vi "UHR-Fleezers Control (host) - 11.0.vi"() -> ()   [LabVIEW 2011] (continued)
            w1289 = FALSE ("Value (Signaling)")
            n927 = case shown="True" w1288 {
              frame False {
              }
              frame True {
                n928 = property on="Sample Channel\nFlow" class="Bool (strict)"("Val(Sgnl)"=FALSE ("Stage Moving")) -> ()  [unwired: 2 in, 2 out]
              }
            }
            n929 = property on="Trap 1 (ON/OFF)" class="Bool (strict)"("Val(Sgnl)"=w1289) -> ()  [unwired: 2 in, 2 out]
            n930 = property on="Trap 2 (ON/OFF)" class="Bool (strict)"("Val(Sgnl)"=w1289) -> ()  [unwired: 2 in, 2 out]
            n931 = call <vilib>:"Beep.vi"() -> ()  [unwired: 3 in, 9 out]
          }
          frame #5 {
            n932 = property on="Move Cap. 2 (ADig Top)" class="Bool (strict)"("Val(Sgnl)"=TRUE ("Value (Signaling)")) -> ()  [unwired: 2 in, 2 out]
            n933 = property on="Tab Control" class="TabCtl (strict)"("Val(Sgnl)"=T4."Status" ("Value (Signaling)")) -> ()  [unwired: 2 in, 2 out]
          }
        }
      }
      event "Dip for Protein": Value Change {
        n934 = event-data() -> ()  [unwired: 1 in, 5 out]
        n935 = case shown="True" "Dip for Protein" {
          tunnel: w1295 -> [_ w1297]
          tunnel: w1294 -> [_ w1296]
          frame False {
          }
          frame True {
            n936 = while {
              tunnel: w1297 -> [w1308]
              tunnel: w1296 -> [w1307]
              i -> [w1302]
              stop <- w1304 stop-if-true
              n937 = Increment(x=w1302) -> (x+1=→"Dip #":i32)
              n938 = flat-sequence {
                tunnel: w1307 -> [w1319]
                tunnel: w1308 -> [w1320]
                tunnel: [w1320] -> w1312
                tunnel: [w1319] -> w1311
                tunnel: [w1313] -> w1298
                tunnel: [w1325] -> w1306
                tunnel: [w1326] -> w1305
                tunnel: w1312 -> [w1327]
                tunnel: w1311 -> [w1328]
                tunnel: [w1323] -> w1299
                tunnel: w1298 -> [w1323]
                tunnel: [w1336] -> w1310
                tunnel: w1306 -> [w1336]
                tunnel: [w1335] -> w1309
                tunnel: w1305 -> [w1335]
                tunnel: [w1332] -> w1303
                tunnel: [w1331] -> w1300
                tunnel: w1299 -> [w1331]
                tunnel: w1309 -> [w1356]
                tunnel: w1310 -> [w1357]
                tunnel: w1303 -> [w1358]
                tunnel: w1300 -> [w1355]
                tunnel: [w1414] -> w1304
                frame #0 {
                  n939 = local read "Trap Pos. FB ON"() -> (w1313:bool)
                  n940 = Compound Arithmetic op=AND("Flow ON\nduring dip?", "FB OFF when \nflow ON", w1313) -> (w1314:bool)
                  n941 = case shown="True" "Move trap \nbefore dip move?" {
                    frame False {
                    }
                    frame True {
                      n942 = property on="Trap Delta (MHz)" class="DigNum (strict)"("Val(Sgnl)"="Dipping Delta (MHz)") -> ()  [unwired: 2 in, 2 out]
                    }
                  }
                  n943 = property on="Green Laser ON/Interlacing" class="Bool (strict)"("Val(Sgnl)"="Green ON\nbefore dip?") -> ()  [unwired: 2 in, 2 out]
                  n944 = property on="Sample Channel\nFlow" class="Bool (strict)"("Val(Sgnl)"="Flow ON\nduring dip?") -> ()  [unwired: 2 in, 2 out]
                  n945 = case shown="True" w1314 {
                    frame False {
                    }
                    frame True {
                      n946 = property on="Trap Pos. FB ON" class="Bool (strict)"("Val(Sgnl)"=FALSE ("Value (Signaling)")) -> ()  [unwired: 2 in, 2 out]
                    }
                  }
                }
                frame #1 {
                  n947 = local read "Saved Stage Positions"() -> (w1330:dbl[][])
                  n948 = local write "Cancel dwell"(FALSE ("Cancel dwell")) -> ()
                  n949 = call "move to saved stage position.vi"("error in"=w1328, "Stage VISA resource name in"=w1327, "Position"="Dip Stage \nPosition", "Saved Stage Positions"=w1330) -> ("VISA resource name out"=w1325:refnum<visa-resource-name>, "error out"=w1326:errorcluster)
                }
                frame #2 {
                  n950 = node-c288() -> (w1334:T21)  [unwired: 4 in]
                  n951 = timed-loop {
                    timing: w1334 -> [_]
                    timing-out: [_] -> w1333
                    tunnel: [w1340] -> w1332
                    i -> [w1337]
                    stop <- w1341 stop-if-true
                    n952 = node-c288() -> ()  [unwired: 1 in, 1 out]
                    n953 = Greater Or Equal?(x=w1337, y="Dip Duration (s)") -> (x >= y?=w1349:bool)
                    n954 = local read "Dip for Protein"() -> (w1342:bool)
                    n955 = local read "Dump Beads"() -> (w1339:bool)
                    n956 = local read "Cancel dwell"() -> (w1348:bool)
                    n957 = local read "Pause dwell"() -> (w1345:bool)
                    n958 = Not(x=w1342) -> (.not. x?=w1347:bool)
                    n959 = Compound Arithmetic op=OR(w1348, w1349, w1347) -> (w1346:bool)
                    n960 = Select(t=FALSE, s=w1345, f=w1346) -> (s? t:f=w1343:bool)
                    n961 = Not(x=w1339) -> (.not. x?=w1338:bool)
                    n962 = node-c288() -> ()  [unwired: 1 in, 1 out]
                    n963 = And(x=w1342, y=w1338) -> (x .and. y?=w1340:bool)
                    n964 = Or(x=w1343, y=w1339) -> (x .or. y?=w1341:bool)
                    "Dip Time (s)" <- w1337
                  }
                  n965 = node-c288(w1333) -> ()  [unwired: 1 out]
                }
                frame #3 {
                  n966 = case shown="True" w1358 {
                    tunnel: w1357 -> [_ w1363]
                    tunnel: w1356 -> [_ w1362]
                    tunnel: w1355 -> [_ w1359]
                    frame False {
                    }
                    frame True {
                      n967 = flat-sequence {
                        tunnel: w1362 -> [w1367]
                        tunnel: w1363 -> [w1368]
                        tunnel: [w1368] -> w1361
                        tunnel: [w1367] -> w1360
                        tunnel: w1359 -> [w1364]
                        tunnel: w1361 -> [w1378]
                        tunnel: w1360 -> [w1377]
                        tunnel: w1359 -> [w1386]
                        frame #0 {
                          n968 = local read "Sample Channel\nFlow"() -> (w1366:bool)
                          n969 = case shown="True" w1366 {
                            tunnel: "Flow ON \nduring return\nfrom dip?" -> [w1369 w1372]
                            tunnel: w1364 -> [_ w1371]
                            frame False {
                              n970 = case shown="True" w1369 {
                                frame False {
                                }
                                frame True {
                                n971 = property on="Sample Channel\nFlow" class="Bool (strict)"("Val(Sgnl)"=TRUE ("Value (Signaling)")) -> ()  [unwired: 2 in, 2 out]
                                }
                              }
                            }
                            frame True {
                              n972 = case shown="False" w1372 {
                                tunnel: w1371 -> [w1373 _]
                                frame False {
                                n973 = property on="Trap Pos. FB ON" class="Bool (strict)"("Val(Sgnl)"=w1373) -> ()  [unwired: 2 in, 2 out]
                                n974 = property on="Sample Channel\nFlow" class="Bool (strict)"("Val(Sgnl)"=FALSE ("Value (Signaling)")) -> ()  [unwired: 2 in, 2 out]
                                }
                                frame True {
                                }
                              }
                            }
                          }
                        }
                        frame #1 {
                          # "For turning on green laser before stage reaches lower spot"
                          n975 = case shown="True" "Green ON\nafter start\nreturn?" {
                            frame False {
                            }
                            frame True {
                              n976 = flat-sequence {
                                frame #0 {
                                n977 = Multiply(x="Green delay after \nstart return (s)", y=1000.0) -> (x*y=w1383:dbl)
                                n978 = Wait (ms)(milliseconds to wait=w1383) -> ()  [unwired: 1 out]
                                }
                                frame #1 {
                                n979 = property on="Green Laser ON/Interlacing" class="Bool (strict)"("Val(Sgnl)"=TRUE ("Value (Signaling)")) -> ()  [unwired: 2 in, 2 out]
                                }
                              }
                            }
                          }
                          n980 = local read "Saved Stage Positions"() -> (w1381:dbl[][])
                          n981 = local write "Cancel dwell"(FALSE ("Cancel dwell")) -> ()
                          n982 = call "move to saved stage position.vi"("error in"=w1377, "Stage VISA resource name in"=w1378, "Position"="Return Stage \nPosition", "Saved Stage Positions"=w1381) -> ("error out"=w1379:errorcluster)  [unwired: 1 out]
                          n983 = local write "Stage Control Serial Error"(w1379) -> ()
                        }
                        frame #2 {
                          n984 = property on="Trap Pos. FB ON" class="Bool (strict)"("Val(Sgnl)"=w1386) -> ()  [unwired: 2 in, 2 out]
                          n985 = case shown="True" "Green ON \nafter return?" {
                            frame False {
                            }
                            frame True {
                              n986 = property on="Green Laser ON/Interlacing" class="Bool (strict)"("Val(Sgnl)"=TRUE ("Value (Signaling)")) -> ()  [unwired: 2 in, 2 out]
                            }
                          }
                          n987 = case shown="True" "Move trap after return?" {
                            frame False {
                            }
                            frame True {
                              n988 = property on="Trap Delta (MHz)" class="DigNum (strict)"("Val(Sgnl)"="Dip Trap Delta 2 (MHz)") -> ()  [unwired: 2 in, 2 out]
                            }
                          }
                          n989 = case shown="True" "Save data after return?" {
                            frame False {
                            }
                            frame True {
                              n990 = property on="Start Saving" class="Bool (strict)"("Val(Sgnl)"=TRUE ("Value (Signaling)")) -> ()  [unwired: 2 in, 2 out]
                            }
                          }
                          n991 = property on="Sample Channel\nFlow" class="Bool (strict)"("Val(Sgnl)"="Flow ON\nduring daq?") -> ()  [unwired: 2 in, 2 out]
                        }
                        frame #3 {
                          n992 = node-c288() -> (w1395:T21)  [unwired: 4 in]
                          n993 = timed-loop {
                            timing: w1395 -> [_]
                            timing-out: [_] -> w1394
                            i -> [w1396]
                            stop <- w1398 stop-if-true
                            n994 = node-c288() -> ()  [unwired: 1 in, 1 out]
                            n995 = local read "Dump Beads"() -> (w1397:bool)
                            n996 = Greater Or Equal?(x=w1396, y="Dwell Duration (s)") -> (x >= y?=w1403:bool)
                            n997 = local read "Dip for Protein"() -> (w1400:bool)
                            n998 = Not(x=w1400) -> (.not. x?=w1399:bool)
                            n999 = Compound Arithmetic op=OR(w1403, "Cancel dwell", w1399) -> (w1402:bool)
                            n1000 = node-c288() -> ()  [unwired: 1 in, 1 out]
                            n1001 = Select(t=FALSE, s="Pause dwell", f=w1402) -> (s? t:f=w1405:bool)
                            n1002 = Or(x=w1405, y=w1397) -> (x .or. y?=w1398:bool)
                            "Dwell Time (s)" <- w1396
                          }
                          n1003 = node-c288(w1394) -> ()  [unwired: 1 out]
                        }
                      }
                    }
                  }
                }
                frame #4 {
                  n1004 = local read "Dip for Protein"() -> (w1415:bool)
                  n1005 = local read "Dump Beads"() -> (w1412:bool)
                  n1006 = local write "Cancel dwell"(FALSE ("Cancel dwell")) -> ()
                  n1007 = Not(x=w1415) -> (.not. x?=w1416:bool)
                  n1008 = Not(x="Cont. Repeat Dipping?") -> (.not. x?=w1418:bool)
                  n1009 = Compound Arithmetic op=OR(w1416, w1418, w1412) -> (w1414:bool)
                }
              }
            }
          }
        }
      }
      event "Profile": Value Change {
        n1010 = event-data() -> ()  [unwired: 1 in, 5 out]
        n1011 = flat-sequence {
          tunnel: w1427 -> [w1430]
          tunnel: w1426 -> [w1438]
          tunnel: [w1432] -> w1425
          tunnel: [w1431] -> w1424
          tunnel: [w1429] -> w1422
          tunnel: [w1428] -> w1419
          tunnel: w1425 -> [w1445]
          tunnel: w1424 -> [w1444]
          tunnel: [w1442] -> w1423
          tunnel: w1422 -> [w1443]
          tunnel: [w1441] -> w1421
          tunnel: [w1440] -> w1420
          tunnel: w1419 -> [w1440]
          tunnel: w1423 -> [w1449]
          tunnel: w1421 -> [w1448]
          tunnel: w1420 -> [w1447]
          frame #0 {
            n1012 = call "Read Stage Position.vi"("error in"=w1438, "VISA resource name in"=w1430) -> ("Current Position"=w1428:cluster{dbl, dbl, dbl}, "error out"=w1431:errorcluster, "VISA resource name out"=w1429:refnum<visa-resource-name>)  [unwired: 1 out]
            "Current Position" <- w1428
            n1013 = local write "Stage Control Serial Error"(w1431) -> ()
            n1014 = Unbundle(w1428) -> (w1435:dbl, w1437:dbl, w1433:dbl)
            n1015 = Add(x=w1437, y="Y change (mm)") -> (x+y=w1434:dbl)
            n1016 = Bundle(w1435, w1434, w1433) -> (w1432:cluster{dbl, dbl, dbl})  [unwired: 1 in]
          }
          frame #1 {
            # "move to new position and start saving"
            n1017 = local write "Stage Moving"(TRUE ("Stage Moving")) -> ()
            n1018 = local write "Start Saving"(TRUE ("Start Saving")) -> ()
            n1019 = call "Set Stage Position.vi"("Position"=w1445, "error in"=w1444, "VISA resource name in"=w1443) -> ("error out"=w1441:errorcluster, "VISA resource name out"=w1442:refnum<visa-resource-name>)  [unwired: 1 out]
          }
          frame #2 {
            # "go back to start"
            n1020 = call "Set Stage Position.vi"("Position"=w1447, "error in"=w1448, "VISA resource name in"=w1449) -> ()  [unwired: 3 out]
          }
          frame #3 {
            # "stop saving"
            n1021 = local write "Stop Saving"(TRUE ("Stop Saving")) -> ()
            n1022 = local write "Stage Moving"(FALSE ("Stage Moving")) -> ()
          }
        }
      }
      event "Move to Position 1", "Move to Position 2", "Move to Position 3", "Move to Position 4", "Move to Position 5", "Lower Ch. Cap.": Value Change {
        n1023 = event-data() -> ()  [unwired: 1 in, 5 out]
        n1024 = Or(x="Move to Position 5", y="Lower Ch. Cap.") -> (x .or. y?=w1455:bool)
        n1025 = Build Array("Move to Position 1", "Move to Position 2", "Move to Position 3", "Move to Position 4", w1455) -> (w1458:bool[])
        n1026 = Boolean Array To Number(Boolean array=w1458) -> (number=w1457:u32)
        n1027 = Logarithm Base 2(1:w1457) -> (0:w1456:dbl)
        n1028 = flat-sequence {
          tunnel: w1456 -> [w1467]
          tunnel: w1453 -> [w1465]
          tunnel: w1452 -> [w1464]
          frame #0 {
            n1029 = local read "Saved Stage Positions"() -> (w1475:dbl[][])
            n1030 = Array Subset(array=w1475, index (row)=w1467, length (row)=1 ("length"), index (col)=1 ("index"), length (col)=3 ("length")) -> (w1472:dbl[][])
            n1031 = Reshape Array(w1472, 3 ("dimension size")) -> (w1470:dbl[])
            n1032 = Array To Cluster(array=w1470) -> (cluster=w1469:cluster{"[0]":dbl, "[1]":dbl, "[2]":dbl})
            n1033 = call "Set Stage Position.vi"("Position"=w1469, "error in"=w1464, "VISA resource name in"=w1465) -> ("error out"=w1468:errorcluster)  [unwired: 2 out]
            n1034 = local write "Stage Moving"(TRUE ("Stage Moving")) -> ()
            n1035 = local write "Stage Control Serial Error"(w1468) -> ()
          }
          frame #1 {
            n1036 = local write "Stage Moving"(FALSE ("Stage Moving")) -> ()
            n1037 = call <vilib>:"Beep.vi"() -> ()  [unwired: 3 in, 9 out]
          }
        }
      }
      event "Got ADig bead": Value Change {
        n1038 = event-data() -> ()  [unwired: 1 in, 5 out]
        n1039 = flat-sequence {
          frame #0 {
            n1040 = local read "Cap 1 Samp Flow ON"() -> (w1479:bool)
            n1041 = case shown="True" w1479 {
              frame False {
              }
              frame True {
                n1042 = property on="Sample Channel\nFlow" class="Bool (strict)"("Val(Sgnl)"=TRUE ("Value (Signaling)")) -> ()  [unwired: 2 in, 2 out]
              }
            }
          }
          frame #1 {
            n1043 = property on="Inject Pump 3" class="Bool (strict)"("Val(Sgnl)"=FALSE ("Value (Signaling)")) -> ()  [unwired: 2 in, 2 out]
          }
          frame #2 {
            n1044 = property on="Move Cap. 1 (DNA Bottom)" class="Bool (strict)"("Val(Sgnl)"=TRUE ("Value (Signaling)")) -> ()  [unwired: 2 in, 2 out]
          }
        }
      }
      event "Force FB Data\nScript": Value Change {
        n1045 = event-data() -> ()  [unwired: 1 in, 5 out]
        n1046 = flat-sequence {
          tunnel: w1488 -> [w1492]
          tunnel: w1489 -> [w1493]
          tunnel: [w1493] -> w1484
          tunnel: [w1492] -> w1483
          tunnel: w1484 -> [w1496]
          tunnel: w1483 -> [w1495]
          tunnel: ["Trap Trig Fl."] -> w1485
          tunnel: [w1521] -> w1486
          tunnel: w1485 -> [w1521]
          tunnel: [w1525] -> w1487
          tunnel: w1486 -> [w1525]
          tunnel: w1487 -> [w1527]
          frame #0 {
            n1047 = property on="Trap Delta (MHz)" class="DigNum (strict)"("Val(Sgnl)"="Trap Delta Before Moving") -> ()  [unwired: 2 in, 2 out]
          }
          frame #1 {
            n1048 = local read "Saved Stage Positions"() -> (w1498:dbl[][])
            n1049 = local write "FB Trap Pos Offset"(0.0 ("FB Trap Pos Offset")) -> ()
            n1050 = property on="Trap Pos. FB Offset Factor" class="DigNum (strict)"("Val(Sgnl)"=i64 0 ("Value (Signaling)")) -> ()  [unwired: 2 in, 2 out]
            n1051 = local write "Stage Moving"(TRUE ("Stage Moving")) -> ()
            n1052 = call "move to saved stage position.vi"("error in"=w1495, "Stage VISA resource name in"=w1496, "Position"="Stage Position To Establish FB", "Saved Stage Positions"=w1498) -> ("error out"=w1494:errorcluster)  [unwired: 1 out]
            n1053 = local write "Stage Control Serial Error"(w1494) -> ()
          }
          frame #2 {
            n1054 = call <vilib>:"Beep.vi"() -> ()  [unwired: 3 in, 9 out]
            n1055 = Multiply(x="Wait (s)", y=u32 1000 ("milliseconds to wait")) -> (x*y=w1504:u32)
            n1056 = property on="Trap Delta (MHz)" class="DigNum (strict)"("Val(Sgnl)"="Starting \nTrap Delta (MHz)") -> ()  [unwired: 2 in, 2 out]
            n1057 = local write "Stage Moving"(FALSE ("Stage Moving")) -> ()
            n1058 = Wait (ms)(milliseconds to wait=w1504) -> ()  [unwired: 1 out]
            n1059 = property on="Tab Control 2" class="TabCtl (strict)"("Val(Sgnl)"=T6."Feedback on Trap Position" ("Value (Signaling)")) -> ()  [unwired: 2 in, 2 out]
            n1060 = property on="Tab Control" class="TabCtl (strict)"("Val(Sgnl)"=T4."Trap Control (RF)" ("Value (Signaling)")) -> ()  [unwired: 2 in, 2 out]
          }
          frame #3 {
            n1061 = property on="Set Reading to\nSetpoint" class="Bool (strict)"("Val(Sgnl)"=TRUE ("Value (Signaling)")) -> ()  [unwired: 2 in, 2 out]
            n1062 = Wait (ms)(milliseconds to wait=u32 500) -> ()  [unwired: 1 out]
          }
          frame #4 {
            n1063 = property on="Trap Pos. FB ON" class="Bool (strict)"("Val(Sgnl)"=TRUE ("Value (Signaling)")) -> ()  [unwired: 2 in, 2 out]
            n1064 = Wait (ms)(milliseconds to wait=u32 250) -> ()  [unwired: 1 out]
          }
          frame #5 {
            n1065 = case shown="False" "Trap Trig Fl." {
              frame False {
                n1066 = case shown="True" "Green ON after FB ON?" {
                  selector: "Green ON after FB ON?" -> [_ w1520]
                  frame False {
                  }
                  frame True {
                    n1067 = property on="Green Laser ON/Interlacing" class="Bool (strict)"("Val(Sgnl)"=w1520) -> ()  [unwired: 2 in, 2 out]
                  }
                }
              }
              frame True {
              }
            }
            n1068 = case shown="True" "Remove Action Offset" {
              tunnel: TRUE ("Value (Signaling)") -> [w1517 w1518]
              frame False {
                n1069 = property on="Remove Unwinding Offset" class="Bool (strict)"("Val(Sgnl)"=w1517) -> ()  [unwired: 2 in, 2 out]
              }
              frame True {
                n1070 = property on="Remove Action Offset" class="Bool (strict)"("Val(Sgnl)"=w1518) -> ()  [unwired: 2 in, 2 out]
              }
            }
            n1071 = Wait (ms)(milliseconds to wait=u32 250) -> ()  [unwired: 1 out]
          }
          frame #6 {
            n1072 = property on="Start Saving" class="Bool (strict)"("Val(Sgnl)"=TRUE ("Value (Signaling)")) -> ()  [unwired: 2 in, 2 out]
            n1073 = Wait (ms)(milliseconds to wait=u32 5000) -> ()  [unwired: 1 out]
          }
          frame #7 {
            w1524 = TRUE ("Value (Signaling)")
            n1074 = property on="Rem fb disp offset" class="Bool (strict)"("Val(Sgnl)"=w1524) -> ()  [unwired: 2 in, 2 out]
            n1075 = property on="Remove Offset" class="Bool (strict)"("Val(Sgnl)"=w1524) -> ()  [unwired: 2 in, 2 out]
            n1076 = Wait (ms)(milliseconds to wait=u32 100) -> ()  [unwired: 1 out]
          }
          frame #8 {
            n1077 = case shown="True" w1527 {
              frame False {
              }
              frame True {
                n1078 = local write "Trap Trig. Fl."(TRUE ("Value (Signaling)")) -> ()
              }
            }
          }
          frame #9 {
            n1079 = case shown="True" "Start dipping after?" {
              frame False {
              }
              frame True {
                n1080 = flat-sequence {
                  frame #0 {
                    n1081 = Multiply(x="Delay before dipping (s)", y=1000.0) -> (x*y=w1531:dbl)
                    n1082 = Wait (ms)(milliseconds to wait=w1531) -> ()  [unwired: 1 out]
                  }
                  frame #1 {
                    n1083 = property on="Dip for Protein" class="Bool (strict)"("Val(Sgnl)"=TRUE ("Value (Signaling)")) -> ()  [unwired: 2 in, 2 out]
                    n1084 = local write "Scripts"(T1."Dipping" ("Scripts")) -> ()
                  }
                }
              }
            }
          }
        }
      }
      event "Fixed Traps Data\nScript": Value Change {
        n1085 = event-data() -> ()  [unwired: 1 in, 5 out]
        n1086 = flat-sequence {
          frame #0 {
            n1087 = case shown="True" "Green ON" {
              frame False {
              }
              frame True {
                n1088 = property on="Green Laser ON/Interlacing" class="Bool (strict)"("Val(Sgnl)"=TRUE) -> ()  [unwired: 2 in, 2 out]
              }
            }
            n1089 = local write "Offset (nm)"(0.0 ("Offset (nm)")) -> ()
            n1090 = property on="Sample Channel\nFlow" class="Bool (strict)"("Val(Sgnl)"=FALSE ("Value (Signaling)")) -> ()  [unwired: 2 in, 2 out]
            n1091 = property on="Trap Delta (MHz)" class="DigNum (strict)"("Val(Sgnl)"="Fixed Traps Trap Delta (MHz)") -> ()  [unwired: 2 in, 2 out]
          }
          frame #1 {
            n1092 = Wait (ms)(milliseconds to wait=u32 1000) -> ()  [unwired: 1 out]
          }
          frame #2 {
            n1093 = local write "Start Saving"(TRUE ("Start Saving")) -> ()
          }
          frame #3 {
            n1094 = local read "Bead Sep. Int. Time (s)"() -> (w1542:dbl)
            n1095 = Multiply(x=w1542, y=1000.0) -> (x*y=w1544:dbl)
            n1096 = Wait (ms)(milliseconds to wait=w1544) -> ()  [unwired: 1 out]
          }
          frame #4 {
            n1097 = property on="Remove Offset" class="Bool (strict)"("Val(Sgnl)"=TRUE ("Value (Signaling)")) -> ()  [unwired: 2 in, 2 out]
          }
          frame #5 {
            n1098 = property on="Dip for Protein" class="Bool (strict)"("Val(Sgnl)"="Start dipping after?") -> ()  [unwired: 2 in, 2 out]
          }
        }
      }
      event "Got DNA bead": Value Change {
        n1099 = event-data() -> ()  [unwired: 1 in, 5 out]
        n1100 = flat-sequence {
          frame #0 {
            n1101 = local read "Daq spot flow on"() -> (w1549:bool)
            n1102 = case shown="True" w1549 {
              frame False {
              }
              frame True {
                n1103 = property on="Sample Channel\nFlow" class="Bool (strict)"("Val(Sgnl)"=TRUE ("Value (Signaling)")) -> ()  [unwired: 2 in, 2 out]
              }
            }
            n1104 = property on="Got DNA bead" class="Bool"("Key Focus"=FALSE) -> ()  [unwired: 2 in, 2 out]
          }
          frame #1 {
            n1105 = property on="Inject Pump 1" class="Bool (strict)"("Val(Sgnl)"=FALSE ("Value (Signaling)")) -> ()  [unwired: 2 in, 2 out]
          }
          frame #2 {
            n1106 = property on="Cal/Data Acq. Spot" class="Bool (strict)"("Val(Sgnl)"=TRUE ("Value (Signaling)")) -> ()  [unwired: 2 in, 2 out]
          }
        }
      }
      event "Take Stepping Data": Value Change {
        n1107 = event-data() -> ()  [unwired: 1 in, 5 out]
        n1108 = local read "Save ave N"() -> (w1561:dbl)
        n1109 = flat-sequence {
          tunnel: w1561 -> [w1563]
          tunnel: [w1563] -> w1556
          tunnel: [w1565] -> w1557
          tunnel: w1556 -> [w1565]
          tunnel: [w1567] -> w1558
          tunnel: w1557 -> [w1567]
          tunnel: [w1570] -> w1559
          tunnel: w1558 -> [w1570]
          tunnel: [w1572] -> w1560
          tunnel: w1559 -> [w1572]
          tunnel: [w1574] -> w1554
          tunnel: w1560 -> [w1574]
          tunnel: w1554 -> [w1577]
          tunnel: [w1577] -> w1553
          tunnel: w1553 -> [w1578]
          tunnel: [w1578] -> w1555
          tunnel: w1555 -> [w1584]
          frame #0 {
            n1110 = property on="Save ave N" class="DigNum (strict)"("Val(Sgnl)"="Save ave factor") -> ()  [unwired: 2 in, 2 out]
          }
          frame #1 {
            n1111 = Wait (ms)(milliseconds to wait=u32 100) -> ()  [unwired: 1 out]
          }
          frame #2 {
            n1112 = local read "Offset 2 Start (MHz)"() -> (w1569:dbl)
            n1113 = property on="Saved AOD Raster Scan Parameter Sets" class="Arr (strict)"("Index Values"=u32[] [2]) -> ()  [unwired: 2 in, 2 out]
            n1114 = property on="Trap Delta (MHz)" class="DigNum (strict)"("Val(Sgnl)"=w1569) -> ()  [unwired: 2 in, 2 out]
          }
          frame #3 {
            n1115 = property on="Load parameters" class="Bool (strict)"("Val(Sgnl)"=TRUE ("Value (Signaling)")) -> ()  [unwired: 2 in, 2 out]
          }
          frame #4 {
            n1116 = Wait (ms)(milliseconds to wait=u32 100) -> ()  [unwired: 1 out]
          }
          frame #5 {
            n1117 = property on="Trap Raster Scan" class="Bool (strict)"("Val(Sgnl)"=TRUE ("Value (Signaling)")) -> ()  [unwired: 2 in, 2 out]
          }
          frame #6 {
            n1118 = Wait (ms)(milliseconds to wait=u32 1000) -> ()  [unwired: 1 out]
          }
          frame #7 {
            n1119 = while {
              stop <- w1581 stop-if-true
              n1120 = local read "Raster Scanning..."() -> (w1583:bool)
              n1121 = local read "Saving..."() -> (w1582:bool)
              n1122 = Not(x=w1582) -> (.not. x?=w1579:bool)
              n1123 = Not(x=w1583) -> (.not. x?=w1580:bool)
              n1124 = And(x=w1580, y=w1579) -> (x .and. y?=w1581:bool)
            }
          }
          frame #8 {
            n1125 = property on="Save ave N" class="DigNum (strict)"("Val(Sgnl)"=w1584) -> ()  [unwired: 2 in, 2 out]
          }
        }
      }
      event "Step Size (nm)": Value Change {
        n1126 = event-data() -> ()  [unwired: 1 in, 5 out]
        n1127 = flat-sequence {
          frame #0 {
            n1128 = property on="Saved AOD Raster Scan Parameter Sets" class="Arr (strict)"("Index Values"=u32[] [1]) -> ()  [unwired: 2 in, 2 out]
          }
          frame #1 {
            n1129 = Multiply(x="N Steps", y="Step Size (nm)") -> (x*y=w1586:dbl)
            n1130 = property on="Scan Speed AOD (nm/s) 2" class="DigNum (strict)"("Value"="Step Size (nm)") -> ()  [unwired: 2 in, 2 out]
            n1131 = property on="Step Size AOD (nm) 2" class="DigNum (strict)"("Value"="Step Size (nm)") -> ()  [unwired: 2 in, 2 out]
            n1132 = property on="Scan Range AOD (nm) 2" class="DigNum (strict)"("Value"=w1586) -> ()  [unwired: 2 in, 2 out]
          }
        }
      }
      event "Take Detection Laser\nImage": Value Change {
        n1133 = event-data() -> ()  [unwired: 1 in, 5 out]
        n1134 = flat-sequence {
          tunnel: [w1614] -> w1604
          tunnel: [w1613] -> w1597
          tunnel: [w1612] -> w1589
          tunnel: [w1617] -> w1605
          tunnel: w1604 -> [w1617]
          tunnel: [w1616] -> w1598
          tunnel: w1597 -> [w1616]
          tunnel: [w1615] -> w1590
          tunnel: w1589 -> [w1615]
          tunnel: [w1621] -> w1606
          tunnel: w1605 -> [w1621]
          tunnel: [w1620] -> w1599
          tunnel: w1598 -> [w1620]
          tunnel: [w1619] -> w1591
          tunnel: w1590 -> [w1619]
          tunnel: [w1627] -> w1607
          tunnel: w1606 -> [w1627]
          tunnel: [w1626] -> w1600
          tunnel: w1599 -> [w1626]
          tunnel: [w1625] -> w1592
          tunnel: w1591 -> [w1625]
          tunnel: [w1631] -> w1608
          tunnel: w1607 -> [w1631]
          tunnel: [w1630] -> w1601
          tunnel: w1600 -> [w1630]
          tunnel: [w1629] -> w1593
          tunnel: w1592 -> [w1629]
          tunnel: [w1635] -> w1609
          tunnel: w1608 -> [w1635]
          tunnel: [w1634] -> w1602
          tunnel: w1601 -> [w1634]
          tunnel: [w1633] -> w1594
          tunnel: w1593 -> [w1633]
          tunnel: [w1639] -> w1610
          tunnel: w1609 -> [w1639]
          tunnel: [w1638] -> w1603
          tunnel: w1602 -> [w1638]
          tunnel: [w1637] -> w1595
          tunnel: w1594 -> [w1637]
          tunnel: w1610 -> [w1645]
          tunnel: w1603 -> [w1644]
          tunnel: [w1642] -> w1596
          tunnel: w1595 -> [w1642]
          tunnel: w1596 -> [w1646]
          frame #0 {
            n1135 = local read "Green Laser ON/Interlacing"() -> (w1614:bool)
            n1136 = local read "Green laser mode"() -> (w1613:enum32{"Laser ON", "Laser OFF", "Interlace"})
            n1137 = local read "Green FB On/Off"() -> (w1612:bool)
          }
          frame #1 {
            n1138 = property on="Green FB On/Off" class="Bool (strict)"("Val(Sgnl)"=FALSE ("Value (Signaling)")) -> ()  [unwired: 2 in, 2 out]
          }
          frame #2 {
            n1139 = property on="Green Laser ON/Interlacing" class="Bool (strict)"("Val(Sgnl)"=TRUE ("Value (Signaling)")) -> ()  [unwired: 2 in, 2 out]
            n1140 = property on="Flip Green Filter" class="Bool (strict)"("Val(Sgnl)"=TRUE ("Value (Signaling)")) -> ()  [unwired: 2 in, 2 out]
            n1141 = property on="Green laser mode" class="RadioBtnsControl (strict)"("Val(Sgnl)"=enum32{"Laser ON", "Laser OFF", "Interlace"}."Laser ON" ("Value (Signaling)")) -> ()  [unwired: 2 in, 2 out]
          }
          frame #3 {
            n1142 = Wait (ms)(milliseconds to wait=u32 500) -> ()  [unwired: 1 out]
          }
          frame #4 {
            n1143 = property on="Confocal Image" class="Bool (strict)"("Val(Sgnl)"=TRUE ("Value (Signaling)")) -> ()  [unwired: 2 in, 2 out]
          }
          frame #5 {
            n1144 = Wait (ms)(milliseconds to wait=u32 2000) -> ()  [unwired: 1 out]
          }
          frame #6 {
            n1145 = while {
              stop <- w1640 stop-if-true
              n1146 = local read "Saving..."() -> (w1641:bool)
              n1147 = Not(x=w1641) -> (.not. x?=w1640:bool)
            }
          }
          frame #7 {
            n1148 = property on="Flip Green Filter" class="Bool (strict)"("Val(Sgnl)"=TRUE ("Value (Signaling)")) -> ()  [unwired: 2 in, 2 out]
            n1149 = property on="Green Laser ON/Interlacing" class="Bool (strict)"("Val(Sgnl)"=w1645) -> ()  [unwired: 2 in, 2 out]
            n1150 = property on="Green laser mode" class="RadioBtnsControl (strict)"("Val(Sgnl)"=w1644) -> ()  [unwired: 2 in, 2 out]
          }
          frame #8 {
            n1151 = property on="Green FB On/Off" class="Bool (strict)"("Val(Sgnl)"=w1646) -> ()  [unwired: 2 in, 2 out]
          }
        }
      }
      event "Stop All": Value Change {
        n1152 = event-data() -> ()  [unwired: 1 in, 5 out]
        n1153 = local read "Stop All"() -> (w1647:bool)
      }
    }
    n1154 = node-c288() -> ()  [unwired: 1 in, 1 out]
  }
  n1155 = node-c288() -> (w94:T21)  [unwired: 4 out]
  n1156 = timed-loop "Control parameters (event loop)" {
    tunnel: w1 -> [w1656]
    shift-right: [w1655] -> _
    shift-left: errorcluster {"status"=FALSE, "code"=0, "source"=""} ("error out") -> [w1654]
    tunnel: [w1653] -> _
    timing: w92 -> [_]
    timing-out: [_] -> w91
    tunnel: w64 -> [w1652]
    tunnel: w5 -> [w1651]
    tunnel: w4 -> [w1650]
    tunnel: w3 -> [w1649]
    tunnel: w2 -> [w1648]
    stop <- w1653 stop-if-true
    n1157 = node-c288() -> ()  [unwired: 2 out]
    n1158 = event shown="[20] \"Green laser mode\", \"Green Laser ON/Interlacing\": Value Change" {
      selector: _ -> [_ _ _ _ _ _ _ _ _ _ _ _ _ _ _ _ _ _ _ _ _ _ _ _ _ _ _ _ _ _ _ _ _ _ _ _ _ _ _ _ _ _ _ _ _ _ _ _ _ _ _ _ _ _ _ _ _ _ _ _ _ _ _ _ _ _ _ _ _ _ _ _ _ _ _]
      dyn-events: _ -> [_ _ _ _ _ _ _ _ _ _ _ _ _ _ _ _ _ _ _ _ _ _ _ _ _ _ _ _ _ _ _ _ _ _ _ _ _ _ _ _ _ _ _ _ _ _ _ _ _ _ _ _ _ _ _ _ _ _ _ _ _ _ _ _ _ _ _ _ _ _ _ _ _ _ _]
      timeout: _ -> [_ _ _ _ _ _ _ _ _ _ _ _ _ _ _ _ _ _ _ _ _ _ _ _ _ _ _ _ _ _ _ _ _ _ _ _ _ _ _ _ _ _ _ _ _ _ _ _ _ _ _ _ _ _ _ _ _ _ _ _ _ _ _ _ _ _ _ _ _ _ _ _ _ _ _]
      tunnel: w1656 -> [w1694 _ _ _ w1732 _ w1754 _ _ _ _ w1820 _ _ w1863 w1869 w1874 w1880 w1916 w1934 w1941 _ w1953 w1957 w1968 w1979 w1990 w2001 w2012 w2023 w2050 w2144 w2151 w2189 _ w2224 w2228 w2239 w2243 w2247 _ w2255 _ _ _ _ _ _ _ _ _ _ _ _ _ _ _ _ _ w2633 _ w2650 _ w2657 w2675 _ w2682 w2690 w2705 w2716 w2722 _ w2731 _ w2750]
      tunnel: [w1693 _ _ _ w1722 _ w1753 _ _ w1785 _ w1799 _ _ w1862 w1865 w1871 w1877 w1915 w1932 w1940 _ w1951 _ w1962 w1973 w1984 w1995 w2006 w2017 w2048 w2142 w2149 w2187 _ w2222 w2226 w2229 w2241 w2245 _ w2253 _ _ _ _ _ _ _ _ _ _ _ _ _ _ _ _ _ w2631 _ _ _ _ w2672 _ _ _ _ _ _ _ _ _ _] -> w1655
      tunnel: w1654 -> [w1692 _ _ _ w1731 _ w1752 _ _ w1785 _ w1819 _ _ w1861 w1864 w1870 w1876 w1914 w1933 w1939 _ w1952 w1956 w1967 w1978 w1989 w2000 w2011 w2022 w2049 w2143 w2150 w2188 _ w2223 w2227 w2238 w2242 w2246 _ w2254 _ _ _ _ _ _ _ _ _ _ _ _ _ _ _ _ _ w2632 _ w2649 _ w2656 w2674 _ w2681 w2689 w2704 w2715 w2721 _ w2730 _ w2749]
      tunnel: [_ _ _ _ _ _ _ _ _ w1784 _ _ _ _ _ _ _ _ _ _ _ _ _ _ _ _ _ _ _ _ _ _ _ _ _ _ _ _ _ _ _ _ _ _ _ _ _ _ _ _ _ _ _ _ _ _ _ _ _ _ _ _ _ _ _ _ _ _ _ _ _ _ _ _ _] -> w1653
      tunnel: [_ _ _ _ _ _ _ "Round T1 X" _ _ _ _ _ _ _ _ _ _ _ _ _ _ _ _ _ _ _ _ _ _ _ _ _ _ _ _ _ _ _ _ _ _ _ _ _ _ _ _ _ _ _ _ _ _ _ _ _ _ _ _ _ _ _ _ _ _ _ _ _ _ _ _ _ _ _] -> _
      tunnel: [_ _ _ "Adjust Scale\nto Mean" _ _ _ _ _ _ _ _ _ _ _ _ _ _ _ _ _ _ "Test ttrig" _ _ _ _ _ _ _ _ _ _ _ _ _ _ _ _ _ _ _ _ _ _ _ _ _ _ "Flush Sample" "Flush Pump 3" "Flush Pump 1" "Clear Volume" _ _ _ _ _ _ _ _ _ _ _ _ _ _ _ _ _ _ _ _ _ _] -> _
      tunnel: [_ _ _ _ _ _ _ _ "Round T2 X" _ "Delayed Interlace Start" _ _ _ _ _ _ _ _ _ _ _ _ _ _ _ _ _ _ _ _ _ _ _ _ _ _ _ _ _ _ _ _ _ _ _ _ _ _ _ _ _ _ _ _ _ _ _ _ _ _ _ _ _ _ _ _ _ _ _ _ _ _ _ _] -> _
      tunnel: w1652 -> [_ _ _ _ _ _ _ _ _ _ _ _ _ _ _ _ _ _ _ _ _ _ _ _ _ _ _ _ _ _ _ _ _ _ _ _ _ _ _ _ _ _ _ _ _ w2412 w2419 w2426 w2431 w2440 _ _ w2546 _ _ _ _ _ _ _ _ _ _ _ _ _ _ _ _ _ _ _ _ _ _]
      tunnel: w1651 -> [_ _ _ _ _ _ _ _ _ _ _ _ _ _ _ _ _ _ _ _ _ _ _ _ _ _ _ _ _ _ _ _ _ _ _ _ _ _ _ _ _ _ _ w2329 _ _ _ _ _ _ w2484 _ _ w2552 _ w2561 _ w2575 _ _ _ _ _ _ _ _ _ _ _ _ _ _ _ _ _]
      tunnel: w1650 -> [_ _ _ _ _ _ _ _ _ _ _ _ _ _ _ _ _ _ _ _ _ _ _ _ _ _ _ _ _ _ _ _ _ _ _ _ _ _ _ _ _ _ _ _ _ _ _ _ _ _ _ _ _ _ _ _ _ _ _ _ _ _ _ _ _ _ _ _ _ _ _ _ _ _ _]
      tunnel: w1649 -> [_ _ _ _ _ _ _ _ _ _ _ _ _ _ _ _ _ _ _ _ _ _ _ _ _ _ _ _ _ _ _ _ _ _ _ _ _ _ _ _ _ _ w2266 _ _ _ _ _ _ _ _ w2514 _ _ w2557 _ w2568 _ w2600 _ _ _ _ _ _ _ _ _ _ _ _ _ _ _ _]
      tunnel: w1648 -> [_ _ _ _ _ _ _ _ _ _ _ _ _ _ _ _ _ _ _ _ _ _ _ _ _ _ _ _ _ _ _ _ _ _ _ _ _ _ _ _ _ _ _ _ _ _ _ _ _ _ _ _ _ _ _ _ _ _ _ _ _ _ _ _ _ _ _ _ _ _ _ _ _ _ _]
      event "AI Count (ticks)", "Sets to FIFO (Traps)", "Save ave N", "FPGA Ave.", "# Samples/channel", "N sets to save": Value Change {
        # "So that if 'Save ave N' is updated, the AOD scanning code updates too."
        n1159 = event-data() -> ()  [unwired: 6 out]
        n1160 = local read "AI Count (ticks)"() -> (w1674:u32)
        n1161 = Boolean To (0,1)(Boolean="Sets to FIFO (Traps)") -> (0, 1=w1684:cluster{"Set 1":i16, "Set 2":i16, "Set 3":i16})
        n1162 = xnode "Read/Write Control"("FPGA VI Reference In"=w1694, "error in"=w1692, "ai count"=w1674, "AI1 Sets to FIFO"="Sets to FIFO (Traps)", "N of AI1 Int Acq Sets"="N Acq Sets (Traps + Fl.)") -> ("error out"=w1693:errorcluster)  [unwired: 1 out]
        n1163 = Cluster To Array(cluster=w1684) -> (array=w1683:i16[])
        n1164 = To Unsigned Long Integer(number=w1683) -> (unsigned 32bit integer=w1663:u32[])
        n1165 = local read "Scan steps (AOD)"() -> (w1685:u64)
        n1166 = Multiply(x=w1674, y="N Acq Sets (Traps + Fl.)") -> (x*y=w1672:u32)
        n1167 = Divide(x=40000000.0, y=w1674) -> (x/y=w1666:dbl)
        "AI rate (Hz)" <- w1666
        "Ave. Rate (Hz)" <- w1666
        n1168 = Add Array Elements(numeric array=w1663) -> (sum=w1675:u32)
        "Trap Sets" <- w1675
        n1169 = Reciprocal(x=w1666) -> (1/x=→"Ave. Period (s)":dbl)
        n1170 = property on="Scan steps (AOD)" class="DigNum (strict)"("Val(Sgnl)"=w1685) -> ()  [unwired: 2 in, 2 out]
        n1171 = Divide(x=w1666, y="N Acq Sets (Traps + Fl.)") -> (x/y=w1689:dbl)
        "Data Rate (Hz)" <- w1689
        n1172 = Reciprocal(x=w1689) -> (1/x=→"Data Period (s)":dbl)
        n1173 = local read "Save ave N"() -> (w1688:dbl)
        n1174 = Divide(x=w1689, y=w1688) -> (x/y=w1687:dbl)
        "Save Data Rate (Hz)" <- w1687
        n1175 = Reciprocal(x=w1687) -> (1/x=→"Save Data Period (s)":dbl)
        n1176 = Multiply(x=w1672, y="# Samples/trap") -> (x*y=w1670:u32)
        "Counts/DMA" <- w1670
        n1177 = property on="Trap Disp. Downsample" class="DigNum (strict)"("Maximum"="# Samples/trap") -> ()  [unwired: 2 in, 2 out]
        n1178 = Multiply(x=w1675, y="# Samples/trap") -> (x*y=w1664:u32)
        "# Samples/channel" <- w1664
        n1179 = Multiply(x=w1664, y=u32 8) -> (x*y=→"Trap AI Elements/DMA read":u32)
        n1180 = local read "APD Int. Count"() -> (w1671:u32)
        n1181 = Multiply(x=w1664, y=u32 3) -> (x*y=→"Trap Pos Elements/DMA read":u32)
        n1182 = Divide(x=w1670, y=w1671) -> (x/y=w1661:dbl)
        "APD Samples/FIFO Acq." <- w1661
        n1183 = Divide(x=w1670, y=40000000.0) -> (x/y=w1668:dbl)
        "DMA Update Period (s)" <- w1668
        n1184 = Multiply(x=2.0, y=w1661) -> (x*y=→"APD Elements/DMA read":dbl)
        n1185 = property on="APD Disp. Downsample" class="DigNum (strict)"("Maximum"=w1661) -> ()  [unwired: 2 in, 2 out]
        n1186 = local read "N sets to save"() -> (w1681:u32)
        n1187 = Multiply(x=w1668, y=w1681) -> (x*y=→"Total Time (s)":dbl)
        "FPGA Averaging" <- FALSE ("FPGA Averaging")
      }
      event "Remove Offset": Value Change {
        n1188 = event-data() -> ()  [unwired: 7 out]
        n1189 = local write "Remove Offset"(FALSE ("Remove Offset")) -> ()
        n1190 = local read "Bead Mean (nm)"() -> (w1696:dbl)
        n1191 = local read "Offset (nm)"() -> (w1697:dbl)
        n1192 = Add(x=w1696, y=w1697) -> (x+y=w1695:dbl)
        n1193 = local write "Offset (nm)"(w1695) -> ()
        n1194 = disable-structure shown="Disabled" {
          frame Disabled {
            n1195 = local read "Bead Mean (nm)"() -> (w1702:dbl)
            n1196 = Add(y=w1702) -> (x=w1701:dbl, x+y=w1700:dbl)
            n1197 = Subtract(x=w1702, y=w1701) -> (x-y=w1699:dbl)
            n1198 = property on="Bead Separation" class="WFChart (strict)"("YScale.Minimum"=w1699) -> ()  [unwired: 2 in, 2 out]
            n1199 = property on="Bead Separation" class="WFChart (strict)"("YScale.Maximum"=w1700) -> ()  [unwired: 2 in, 2 out]
          }
          frame Enabled {
          }
        }
      }
      event "Detector Type": Value Change {
        n1200 = event-data() -> ()  [unwired: 7 out]
        n1201 = local read "AI labels"() -> (w1703:string[])
        n1202 = property on="High Res. Display" class="Ring (strict)"("Strings []"=w1703) -> ()  [unwired: 2 in, 2 out]
        n1203 = Build Array (concatenate)(w1703, "none") -> (w1704:string[])
        n1204 = property on="FFT 1 Choice 1" class="Ring (strict)"("Strings []"=w1704) -> ()  [unwired: 2 in, 2 out]
        n1205 = property on="FFT 1 Choice 2" class="Ring (strict)"("Strings []"=w1704) -> ()  [unwired: 2 in, 2 out]
        n1206 = property on="FFT 2 Choice 1" class="Ring (strict)"("Strings []"=w1704) -> ()  [unwired: 2 in, 2 out]
        n1207 = property on="FFT 2 Choice 2" class="Ring (strict)"("Strings []"=w1704) -> ()  [unwired: 2 in, 2 out]
        n1208 = Bundle("APD 1", "APD 2") -> (w1707:cluster{string, string})  [unwired: 1 out]
        n1209 = Cluster To Array(cluster=w1707) -> (array=w1705:string[])
        n1210 = Build Array (concatenate)(w1705, w1704) -> (w1709:string[])
        n1211 = Array Size(array=w1709) -> (size(s)=w1710:i32)
        n1212 = property on="Signals to Plot" class="LstBox (strict)"("Item Names"=w1709) -> ()  [unwired: 2 in, 2 out]
        n1213 = property on="Signals to Plot" class="LstBox (strict)"("Number of Rows"=w1710) -> ()  [unwired: 2 in, 2 out]
        n1214 = property on="All Signals" class="WFChart (strict)"("LegNumRows"=w1710) -> ()  [unwired: 2 in, 2 out]
      }
      event "Adjust Scale\nto Mean": Value Change {
        n1215 = event-data() -> ()  [unwired: 7 out]
        n1216 = local read "APD 1 Rate (Hz)"() -> (w1719:dbl)
        n1217 = Multiply(x=1000.0, y="Above (kHz)") -> (x*y=w1717:dbl)
        n1218 = Multiply(x=1000.0, y="Below (kHz)") -> (x*y=w1715:dbl)
        n1219 = Add(x=w1717, y=w1719) -> (x+y=w1712:dbl)
        n1220 = Subtract(x=w1719, y=w1715) -> (x-y=w1713:dbl)
        n1221 = property on="APD Chart" class="WFChart (strict)"("YScale.Minimum"=w1713) -> ()  [unwired: 2 in, 2 out]
        n1222 = property on="APD Chart" class="WFChart (strict)"("YScale.Maximum"=w1712) -> ()  [unwired: 2 in, 2 out]
      }
      event "Phase adj. (AI1)", "+ phase (AI1)", "- phase (AI1)": Value Change {
        n1223 = event-data() -> ()  [unwired: 7 out]
        n1224 = Negate(x="Phase adj. (AI1)") -> (-x=w1729:i16)
        n1225 = Select(t=w1729, s="- phase (AI1)", f="Phase adj. (AI1)") -> (s? t:f=w1728:i16)
        n1226 = xnode "Read/Write Control"("FPGA VI Reference In"=w1732, "error in"=w1731, "Phase count adjustment"=w1728) -> ("FPGA VI Reference Out"=w1727:T19, "error out"=w1726:errorcluster)
        n1227 = Or(x="- phase (AI1)", y="+ phase (AI1)") -> (x .or. y?=w1723:bool)
        n1228 = xnode "Read/Write Control"("FPGA VI Reference In"=w1727, "error in"=w1726, "+ phase"=w1723) -> ("error out"=w1722:errorcluster)  [unwired: 1 out]
      }
      event "Signals to Plot": Double Click {
        w1735 = u32 9868950 ("Color Box")
        n1229 = event-data() -> ("Row"=w1737:i32)  [unwired: 9 out]
        n1230 = property on="All Signals" class="WFChart (strict)"("Active Plot"=w1737) -> (error out=w1748:errorcluster)  [unwired: 2 in, 1 out]
        n1231 = property on="All Signals" class="WFChart (strict)" props=["Plot", "Visible?", "Plot", "Plot Color"](error in=w1748) -> (error out=w1747:errorcluster, "Plot.Visible?"=w1746:bool)  [unwired: 1 in, 2 out]
        n1232 = Select(t=FALSE ("Plot.Visible"), s=w1746, f=TRUE ("Plot.Visible")) -> (s? t:f=w1741:bool)
        n1233 = property on="All Signals" class="WFChart (strict)"(error in=w1747, "Plot.Visible?"=w1741) -> (error out=w1743:errorcluster)  [unwired: 1 in, 1 out]
        n1234 = property on="All Signals" class="WFChart (strict)"(error in=w1743) -> (error out=w1738:errorcluster, "Plot.Plot Color"=w1742:u32)  [unwired: 1 in, 1 out]
        n1235 = property on="Signals to Plot" class="LstBox (strict)"(error in=w1738, "Active Row"=w1737) -> (error out=w1736:errorcluster)  [unwired: 1 in, 1 out]
        n1236 = Select(t=w1742, s=w1741, f=u32 0) -> (s? t:f=w1739:u32)
        n1237 = property on="Signals to Plot" class="LstBox (strict)"(error in=w1736, "CellFontColor"=w1739, "SelColor"=w1735, "CellBG"=w1735, "CellFontSize"=u32 20 ("Active Row:Cell Font:Size"), "CellFontBold"=TRUE ("Active Row:Cell Font:Bold")) -> ()  [unwired: 1 in, 2 out]
      }
      event "BD 1 Frequency 1 (MHz)", "BD 1 Frequency 2 (MHz)", "BD 1 Frequency 3 (MHz)", "BD 2 Frequency 1 (MHz)", "BD 2 Frequency 2 (MHz)", "BD 2 Frequency 3 (MHz)", "Trap Delta (MHz)": Value Change {
        n1238 = event-data() -> ("CtlRef"=w1751:refnum<vi>)  [unwired: 6 out]
        n1239 = control-ref of="Trap Delta (MHz)"() -> (w1750:refnum<vi>)
        n1240 = Equal?(x=w1750, y=w1751) -> (x = y?=w1749:bool)
        n1241 = case shown="False" "Oscillate Set 1" {
          tunnel: w1754 -> [w1774 _]
          tunnel: [w1773 w1777] -> w1753
          tunnel: w1752 -> [w1772 w1777]
          tunnel: w1749 -> [w1757 _]
          frame False {
            n1242 = local read "BD 1 Frequency 2 (MHz)"() -> (w1761:dbl)
            n1243 = local read "BD 1 Frequency 1 (MHz)"() -> (w1759:dbl)
            n1244 = Subtract(x=w1761, y="Trap Delta (MHz)") -> (x-y=w1758:dbl)
            n1245 = Select(t=w1758, s=w1757, f=w1759) -> (s? t:f=w1756:dbl)
            n1246 = local read "Y RF Frequency Limits (MHz)"() -> (w1762:T16)
            n1247 = local read "X RF Frequency Limits (MHz)"() -> (w1763:T16)
            n1248 = local read "BD 1 Frequency 3 (MHz)"() -> (w1775:dbl)
            n1249 = local write "BD 1 Frequency 1 (MHz)"(w1756) -> ()
            n1250 = local read "BD 2 Frequency 1 (MHz)"() -> (w1766:dbl)
            n1251 = local read "BD 2 Frequency 2 (MHz)"() -> (w1765:dbl)
            n1252 = local read "BD 2 Frequency 3 (MHz)"() -> (w1776:dbl)
            n1253 = call "set RF board frequency - interlace.vi"("Board 2 Frequency Limits"=w1762, "Board 1 Frequency Limits"=w1763, "error in"=w1772, "FPGA VI Reference In"=w1774, "Board 2 Frequency 3 (MHz)"=w1776, "Board 1 Frequency 3 (MHz)"=w1775, "Board 2 Frequency 2 (MHz)"=w1765, "Board 2 Frequency 1 (MHz)"=w1766, "Board 1 Frequency 2 (MHz)"=w1761, "Board 1 Frequency 1  (MHz)"=w1756) -> ("error out"=w1773:errorcluster)  [unwired: 1 out]
            n1254 = Subtract(x=w1766, y=w1765) -> (x-y=w1770:dbl)
            n1255 = Subtract(x=w1756, y=w1761) -> (x-y=w1771:dbl)
            n1256 = Square(x=w1770) -> (x^2=w1768:dbl)
            n1257 = Square(x=w1771) -> (x^2=w1769:dbl)
            n1258 = Add(x=w1769, y=w1768) -> (x+y=w1767:dbl)
            n1259 = Square Root(x=w1767) -> (sqrt(x)=w1764:dbl)
            n1260 = local write "Trap Delta (MHz)"(w1764) -> ()
            n1261 = property on="Initial delta (MHz)" class="DigNum (strict)"("Val(Sgnl)"=w1764) -> ()  [unwired: 2 in, 2 out]
          }
          frame True {
          }
        }
      }
      event "Round T1 X": Value Change {
        n1262 = event-data() -> ()  [unwired: 7 out]
        n1263 = local read "BD 1 Frequency 1 (MHz)"() -> (w1780:dbl)
        n1264 = Round To Nearest(number=w1780) -> (nearest integer value=w1779:dbl)
        n1265 = property on="BD 1 Frequency 1 (MHz)" class="DigNum (strict)"("Val(Sgnl)"=w1779) -> ()  [unwired: 2 in, 2 out]
      }
      event "Round T2 X": Value Change {
        n1266 = event-data() -> ()  [unwired: 7 out]
        n1267 = local read "BD 1 Frequency 2 (MHz)"() -> (w1782:dbl)
        n1268 = Round To Nearest(number=w1782) -> (nearest integer value=w1781:dbl)
        n1269 = property on="BD 1 Frequency 2 (MHz)" class="DigNum (strict)"("Val(Sgnl)"=w1781) -> ()  [unwired: 2 in, 2 out]
      }
      event "Stop All": Value Change {
        n1270 = event-data() -> ()  [unwired: 7 out]
        n1271 = local read "Stop All"() -> (w1784:bool)
      }
      event "Delayed Interlace Start": Value Change {
        n1272 = event-data() -> ()  [unwired: 7 out]
        n1273 = flat-sequence {
          frame #0 {
            n1274 = Multiply(x="Delay to Interlace (s)", y=1000.0) -> (x*y=w1787:dbl)
            n1275 = Wait (ms)(milliseconds to wait=w1787) -> ()  [unwired: 1 out]
          }
          frame #1 {
            n1276 = property on="Green laser mode" class="RadioBtnsControl (strict)"("Val(Sgnl)"=enum32{"Laser ON", "Laser OFF", "Interlace"}."Interlace" ("Value (Signaling)")) -> ()  [unwired: 2 in, 2 out]
          }
        }
      }
      event "BD 1 Amplitude 1 (%)", "BD 1 Amplitude 2 (%)", "BD 1 Amplitude 3 (%)", "BD 2 Amplitude 1 (%)", "BD 2 Amplitude 2 (%)", "BD 2 Amplitude 3 (%)", "Trap 1 ON", "Trap 2 ON", "Trap 3 ON", "Feedback On/Off", "All FB On/Off": Value Change {
        w1811 = i16 1 ("f")
        n1277 = event-data() -> ()  [unwired: 7 out]
        n1278 = local write "Trap 1 (ON/OFF)"("Trap 1 ON") -> ()
        n1279 = local write "Trap 2 (ON/OFF)"("Trap 2 ON") -> ()
        n1280 = Boolean To (0,1)(Boolean="Trap 3 ON") -> (0, 1=w1812:i16)
        n1281 = Boolean To (0,1)(Boolean="Trap 1 ON") -> (0, 1=w1813:i16)
        n1282 = Boolean To (0,1)(Boolean="Trap 2 ON") -> (0, 1=w1814:i16)
        n1283 = Select(t=w1814, s="Trap ON/OFF X or Y Amp?", f=w1811) -> (s? t:f=w1809:i16)
        n1284 = Select(t=w1813, s="Trap ON/OFF X or Y Amp?", f=w1811) -> (s? t:f=w1810:i16)
        n1285 = Select(t=w1812, s="Trap ON/OFF X or Y Amp?", f=w1811) -> (s? t:f=w1808:i16)
        n1286 = Select(t=w1811, s="Trap ON/OFF X or Y Amp?", f=w1814) -> (s? t:f=w1806:i16)
        n1287 = Select(t=w1811, s="Trap ON/OFF X or Y Amp?", f=w1813) -> (s? t:f=w1807:i16)
        n1288 = Select(t=w1811, s="Trap ON/OFF X or Y Amp?", f=w1812) -> (s? t:f=w1805:i16)
        n1289 = And(x="All FB On/Off", y="Feedback On/Off") -> (x .and. y?=w1803:cluster{"Set 1":bool, "Set 2":bool})
        n1290 = local read "BD 1 Amplitude 1 (%)"() -> (w1823:dbl)
        n1291 = local read "BD 1 Amplitude 2 (%)"() -> (w1822:dbl)
        n1292 = local read "BD 1 Amplitude 3 (%)"() -> (w1821:dbl)
        n1293 = Unbundle By Name(w1803) -> ("Set 1"=w1798:bool, "Set 2"=w1795:bool)
        n1294 = local read "Y RF Amplitude Limits (%)"() -> (w1791:T16)
        n1295 = local read "X RF Amplitude Limits (%)"() -> (w1792:T16)
        n1296 = local read "BD 2 Amplitude 1 (%)"() -> (w1824:dbl)
        n1297 = local read "BD 2 Amplitude 2 (%)"() -> (w1825:dbl)
        n1298 = local read "BD 2 Amplitude 3 (%)"() -> (w1826:dbl)
        n1299 = And(x="Trap 2 ON", y=w1795) -> (x .and. y?=w1793:bool)
        n1300 = And(x="Trap 1 ON", y=w1798) -> (x .and. y?=w1796:bool)
        n1301 = Multiply(x=w1810, y=w1823) -> (x*y=w1818:dbl)
        n1302 = Multiply(x=w1822, y=w1809) -> (x*y=w1816:dbl)
        n1303 = Multiply(x=w1821, y=w1808) -> (x*y=w1817:dbl)
        n1304 = Multiply(x=w1824, y=w1807) -> (x*y=w1827:dbl)
        n1305 = Multiply(x=w1825, y=w1806) -> (x*y=w1828:dbl)
        n1306 = Multiply(x=w1826, y=w1805) -> (x*y=w1829:dbl)
        n1307 = call "set RF board amplitude - interlace.vi"("Board 2 Amplitude Limits"=w1791, "Board 1 Amplitude Limits"=w1792, "error in"=w1819, "FPGA VI Reference In"=w1820, "Board 2 Amplitude 3 (%)"=w1829, "Board 1 Amplitude 3 (%)"=w1817, "Board 2 Amplitude 2 (%)"=w1828, "Board 2 Amplitude 1 (%)"=w1827, "Board 1 Amplitude 2 (%)"=w1816, "Board 1 Amplitude 1 (%)"=w1818) -> ("error out"=w1800:errorcluster, "FPGA VI Reference Out"=w1801:T19)
        n1308 = xnode "Read/Write Control"("FPGA VI Reference In"=w1801, "error in"=w1800, "FB On/Off Set 1"=w1796, "FB On/Off Set 2"=w1793) -> ("error out"=w1799:errorcluster)  [unwired: 1 out]
      }
      event "Load parameters": Value Change {
        n1309 = event-data() -> ()  [unwired: 7 out]
        n1310 = property on="Saved AOD Raster Scan Parameter Sets" class="Arr (strict)"() -> ("Index Values"=w1840:u32[])  [unwired: 2 in, 2 out]
        n1311 = Index Array(array=w1840, index=0) -> (element=w1837:u32)
        n1312 = local write "Load parameters"(FALSE ("Load parameters")) -> ()
        n1313 = Index Array(array="Saved AOD Raster Scan Parameter Sets", index=w1837) -> (element=w1836:T26)
        n1314 = Unbundle By Name(w1836) -> ("Scan Range AOD (nm) 2"=w1835:dbl, "Step Size AOD (nm) 2"=w1834:dbl, "Scan Speed AOD (nm/s) 2"=w1833:dbl, "Number of scans (AOD) 2"=w1832:u16)
        n1315 = flat-sequence {
          tunnel: w1835 -> [w1843]
          tunnel: w1834 -> [w1842]
          tunnel: w1833 -> [w1841]
          tunnel: w1832 -> [w1844]
          frame #0 {
            n1316 = local write "Scan Speed (nm/s)"(w1841) -> ()
            n1317 = local write "Scan Range (nm)"(w1843) -> ()
            n1318 = local write "Step Size (nm)"(w1842) -> ()
          }
          frame #1 {
            n1319 = property on="Number of F/B Scans (AOD)" class="DigNum (strict)"("Val(Sgnl)"=w1844) -> ()  [unwired: 2 in, 2 out]
          }
        }
      }
      event "Trap 1 (ON/OFF)", "Trap 2 (ON/OFF)": Value Change {
        n1320 = event-data() -> ()  [unwired: 7 out]
        n1321 = property on="Trap 2 ON" class="Bool (strict)"("Val(Sgnl)"="Trap 2 (ON/OFF)") -> ()  [unwired: 2 in, 2 out]
        n1322 = property on="Trap 1 ON" class="Bool (strict)"("Val(Sgnl)"="Trap 1 (ON/OFF)") -> ()  [unwired: 2 in, 2 out]
      }
      event "DIO count 1 (ticks)", "DIO count 2 (ticks)", "DIO count 3 (ticks)", "Interlace", "Number Interlace Sets", "Not-Interlacing Set": Value Change {
        n1323 = event-data() -> ()  [unwired: 7 out]
        n1324 = local read "DIO count 3 (ticks)"() -> (w1857:u32)
        n1325 = local read "DIO count 1 (ticks)"() -> (w1859:u32)
        n1326 = local read "DIO count 2 (ticks)"() -> (w1858:u32)
        n1327 = To Unsigned Byte Integer(number="Not-Interlacing Set") -> (unsigned 8bit integer=w1848:u8)
        n1328 = Add(x=w1848, y=u8 1) -> (x+y=w1852:u8)
        n1329 = xnode "Read/Write Control"("FPGA VI Reference In"=w1863, "error in"=w1861, "DIO count 1 (ticks)"=w1859, "DIO count 2 (ticks)"=w1858, "DIO count 3 (ticks)"=w1857, "Interlace ON/OFF"="Interlace", "Number Interlace Cycles"="Number Interlace Sets", "Interlace Off Parameters"=w1852) -> ("error out"=w1862:errorcluster)  [unwired: 1 out]
        n1330 = Build Array(w1859, w1858, w1857) -> (w1850:u32[])
        n1331 = Split 1D Array(array=w1850, index="Number Interlace Sets") -> (first subarray=w1860:u32[])  [unwired: 1 out]
        n1332 = Index Array(array=w1850, index=w1848) -> (element=w1849:u32)
        n1333 = Add Array Elements(numeric array=w1860) -> (sum=w1854:u32)
        n1334 = Select(t=w1854, s="Interlace", f=w1849) -> (s? t:f=→"Total Counts (ticks)":u32)
      }
      event "Reset Feedback": Value Change {
        n1335 = event-data() -> ()  [unwired: 7 out]
        n1336 = Unbundle By Name("Reset Feedback") -> ("Set 1"=w1867:bool, "Set 2"=w1866:bool)
        n1337 = xnode "Read/Write Control"("FPGA VI Reference In"=w1869, "error in"=w1864, "FB Reset Set 1"=w1867, "FB Reset Set 2"=w1866) -> ("error out"=w1865:errorcluster)  [unwired: 1 out]
      }
      event "PID Gains": Value Change {
        n1338 = event-data() -> ()  [unwired: 7 out]
        n1339 = Unbundle By Name("PID Gains") -> ("Set 1"=w1873:T14, "Set 2"=w1872:T14)
        n1340 = xnode "Read/Write Control"("FPGA VI Reference In"=w1874, "error in"=w1870, "FB Gains Set 1"=w1873, "FB Gains Set 2"=w1872) -> ("error out"=w1871:errorcluster)  [unwired: 1 out]
      }
      event "AI2 to Setpoint", "Setpoints (V)": Value Change {
        n1341 = event-data() -> ()  [unwired: 7 out]
        n1342 = xnode "Read/Write Control"("FPGA VI Reference In"=w1880, "error in"=w1876) -> ("FPGA VI Reference Out"=w1879:T19, "error out"=w1878:errorcluster, "AI2 Y Sum Set 1"=w1887:i16, "AI2 Y Sum Set 2"=w1886:i16)
        n1343 = Cluster To Array(cluster="AI2 to Setpoint") -> (array=w1890:bool[])
        n1344 = local read "AI2 (V)"() -> (w1888:cluster{"Set 1":dbl, "Set 2":dbl})
        n1345 = Or Array Elements(Boolean array=w1890) -> (logical OR=w1891:bool)
        n1346 = Bundle By Name(cluster=w1888, "Set 1"=w1887, "Set 2"=w1886) -> (w1885:cluster{"Set 1":dbl, "Set 2":dbl})
        n1347 = Divide(x=w1885, y=3276.7) -> (x/y=w1884:cluster{"Set 1":dbl, "Set 2":dbl})
        "AI2 (V)" <- w1884
        n1348 = case shown="True" w1891 {
          tunnel: [w1894 w1911] -> w1883
          tunnel: "AI2 to Setpoint" -> [_ w1907]
          tunnel: "Setpoints (V)" -> [w1895 w1910]
          tunnel: w1884 -> [_ w1904]
          frame False {
            n1349 = Multiply(x=3276.7, y=w1895) -> (x*y=w1896:cluster{"Set 1":dbl, "Set 2":dbl})
            n1350 = To Word Integer(number=w1896) -> (16bit integer=w1894:cluster{"Set 1":i16, "Set 2":i16})
          }
          frame True {
            n1351 = Unbundle By Name(w1904) -> ("Set 1"=w1903:dbl, "Set 2"=w1902:dbl)
            n1352 = Unbundle By Name(w1910) -> ("Set 1"=w1909:dbl, "Set 2"=w1908:dbl)
            n1353 = Unbundle By Name(w1907) -> ("Set 1"=w1906:bool, "Set 2"=w1905:bool)
            n1354 = Select(t=w1903, s=w1906, f=w1909) -> (s? t:f=w1901:dbl)
            n1355 = Select(t=w1902, s=w1905, f=w1908) -> (s? t:f=w1900:dbl)
            n1356 = Bundle By Name(cluster=w1910, "Set 1"=w1901, "Set 2"=w1900) -> (w1898:cluster{"Set 1":dbl, "Set 2":dbl})
            n1357 = local write "Setpoints (V)"(w1898) -> ()
